vi "Find Start Stop.vi"(10 "Boolean array":bool[](array[boolean])) -> (1 "Stop indexes":i32[](array[numeric]), 2 "Start indexes":i32[](array[numeric]))   [LabVIEW 2009]
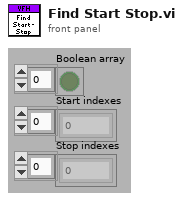
[diagram p1: front panel]
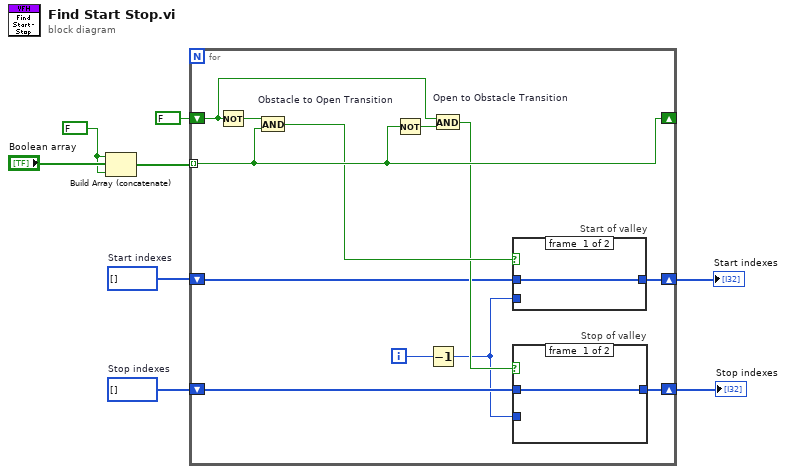
[diagram p0: block diagram]
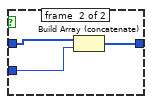
[diagram p2: hidden frame]
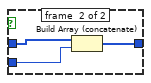
[diagram p3: hidden frame]
diagram:
  w2 = FALSE
  w6 = i32[] []  # Stop indexes
  w7 = i32[] []  # Start indexes
  n1 = Build Array (concatenate)(w2, "Boolean array", w2) -> (w1:bool[])
  n2 = for {
    tunnel: w1 -> [w18] mode=indexing
    shift-right: [w18] -> _
    shift-left: FALSE -> [w17]
    shift-right: [w12] -> w5
    shift-left: w7 -> [w14]
    shift-right: [w11] -> w4
    shift-left: w6 -> [w13]
    i -> [w10]
    n3 = Not(x=w17) -> (.not. x?=w20:bool)
    n4 = And "Obstacle to Open Transition"(x=w20, y=w18) -> (x .and. y?=w16:bool)
    n5 = Not(x=w18) -> (.not. x?=w19:bool)
    n6 = Decrement(x=w10) -> (x-1=w9:i32)
    n7 = And "Open to Obstacle Transition"(x=w17, y=w19) -> (x .and. y?=w15:bool)
    n8 = case "Start of valley" shown="True" w16 {
      tunnel: w14 -> [w25 w28]
      tunnel: w9 -> [_ w27]
      tunnel: [w25 w26] -> w12
      frame #0 {
      }
      frame #1 {
        n9 = Build Array (concatenate)(w28, w27) -> (w26:i32[])
      }
    }
    n10 = case "Stop of valley" shown="True" w15 {
      tunnel: w13 -> [w21 w24]
      tunnel: w9 -> [_ w23]
      tunnel: [w21 w22] -> w11
      frame #0 {
      }
      frame #1 {
        n11 = Build Array (concatenate)(w24, w23) -> (w22:i32[])
      }
    }
  }
  "Start indexes" <- w5
  "Stop indexes" <- w4
